vi "Main.vi"(11 "Module Admin":refnum<class "Delacor_lib_QMH_Module Admin.lvclass">) -> ()   [LabVIEW 2024, in "SingletonSubpanel.lvlib"]
doc: "This template is based off of the Queued Message Handler design pattern and the Queued Message Handler project template that ships with LabVIEW.\n\nThe main difference is that the queue is private to this module and communication between modules is performed via Broadcast and Request events.\n\nRequest events are wrapped in public API methods and are handled in the Event Handling Loop (EHL) of this VI. Any module can register for Broadcast events sent by this module. The EHL generates messages based on user interface actions.\n\nThe Message Handling Loop (MHL) processes messages generated by the EHL, or by other messages. The messages are string values, so new messages can be added easily to the Message Cases case structure in the MHL. Each message cluster can also provide an optional value for Message Data, which is a variant that can be converted to whatever message-specific data is required.\n_____\nBased on DQMH Dev Tools: Project Template 7.1.0.1503."
uses:
  SingletonSubpanel.lvlib
  <vilib>/Delacor/Delacor QMH/Libraries/Module Admin_class/Delacor_lib_QMH_Module Admin.lvclass
  Module Data--cluster.ctl
  <vilib>/Delacor/Delacor QMH/Libraries/Message Queue_class/Delacor_lib_QMH_Message Queue.lvclass/Delacor_lib_QMH_Message Queue.ctl
  Stop Argument--cluster.ctl
  <vilib>/Delacor/Delacor QMH/Libraries/Module Admin_class/Delacor_lib_QMH_Module Admin.lvclass/Delacor_lib_QMH_Module Admin.ctl
  Draw FP in Subpanel Argument--cluster.ctl
  Remove From Subpanel Argument--cluster.ctl
  <vilib>/Utility/miscctls.llb/LVPointTypeDef.ctl
  <vilib>/Delacor/Delacor QMH/Libraries/Message Queue_class/Delacor_lib_QMH_Enqueue Message (Single).vi
  <vilib>/Delacor/Delacor QMH/Libraries/Module Admin_class/Delacor_lib_QMH_Get External Launch.vi
  <vilib>/Delacor/Delacor QMH/Libraries/Message Queue_class/Delacor_lib_QMH_Message Queue.lvclass
panel:
  out "error out":errorcluster
  out "Status":string
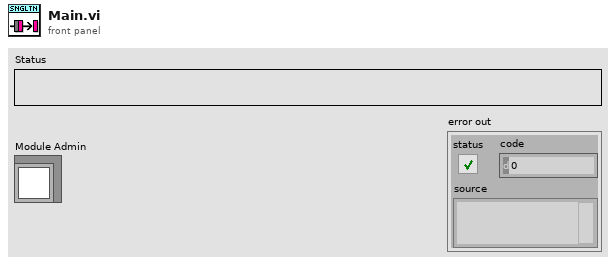
[diagram p1: front panel]
types:
  T1 = typedef "SingletonSubpanel.lvlib/Request Events--cluster.ctl" = cluster{"Stop Module":refnum<user-event>, "Show Panel":refnum<user-event>, "Hide Panel":refnum<user-event>, "Get Module Execution Status":refnum<user-event>, "Show Diagram":refnum<user-event>, "Draw FP in Subpanel":refnum<user-event>, "Remove From Subpanel":refnum<user-event>}
  T2 = typedef "SingletonSubpanel.lvlib/Module Data--cluster.ctl" = cluster{"Status":string, "Sub Panel":refnum<vi>}
  T3 = enum32{"invalid lock state", "Not Locked", "Locked (No Password)", "Password-protected"}
  T4 = typedef "SingletonSubpanel.lvlib/Stop Argument--cluster.ctl" = cluster{"Origin":string, "Exit via Stop Module Req?":bool, "Wait for Module to stop?":bool}
  T5 = typedef "SingletonSubpanel.lvlib/Draw FP in Subpanel Argument--cluster.ctl" = cluster{"Sub Panel":refnum<vi>}
  T6 = typedef "SingletonSubpanel.lvlib/Remove From Subpanel Argument--cluster.ctl" = cluster{"Boolean":bool}
  T7 = typedef "LVPointTypeDef.ctl" = cluster{"Horizontal":i16, "Vertical":i16}
  T8 = enum32{"Invalid", "Standard", "Closed", "Hidden", "Minimized", "Maximized"}
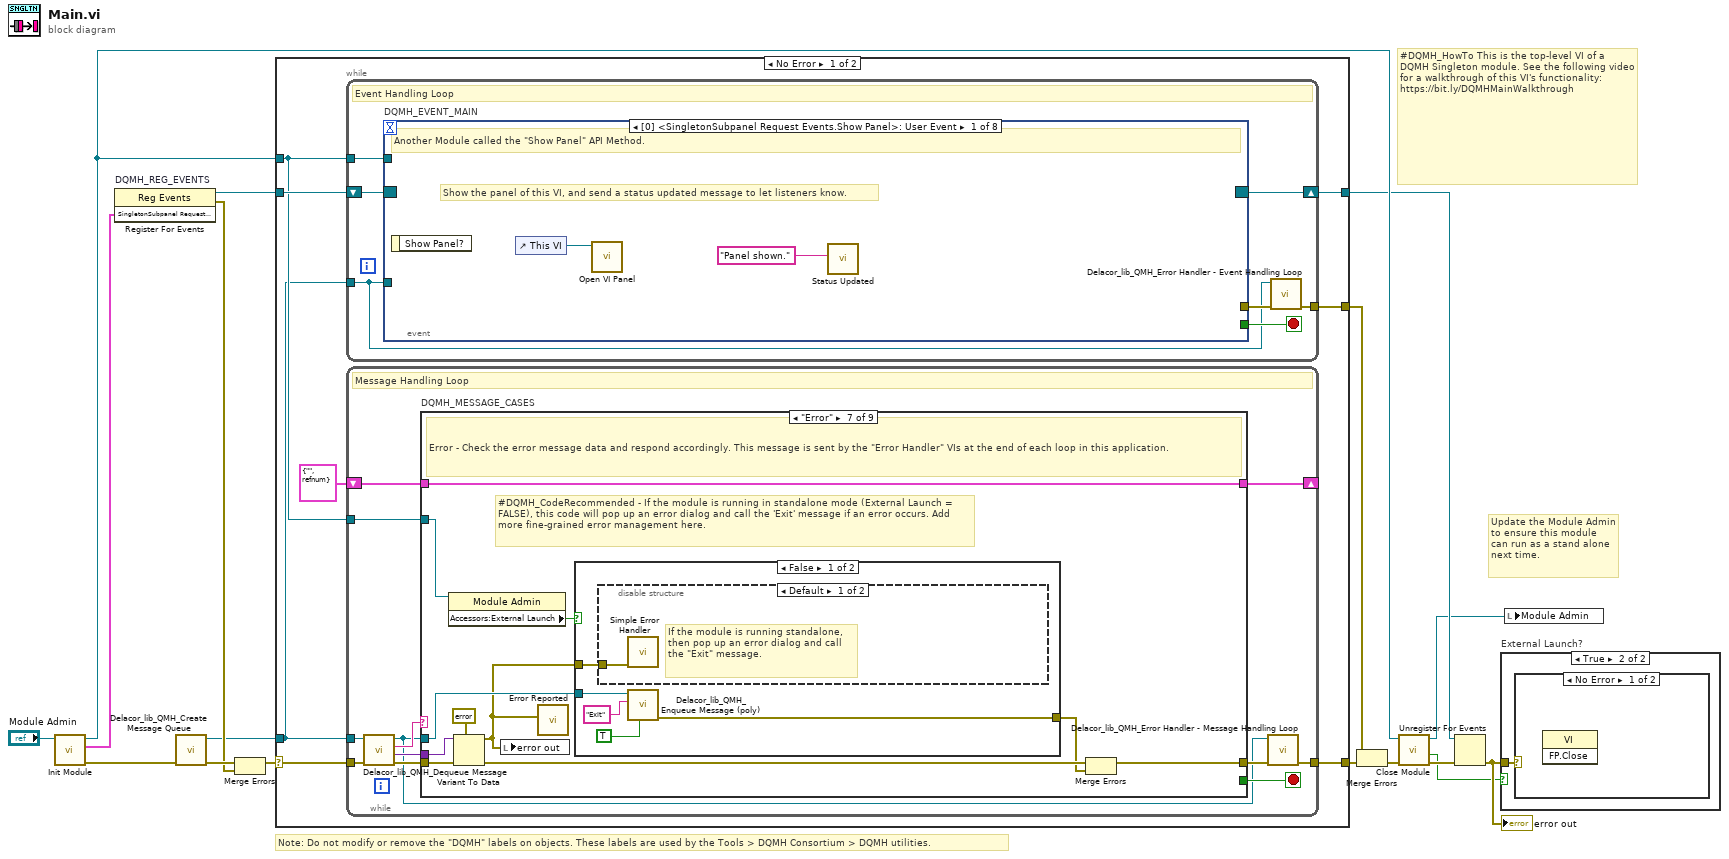
[diagram p0: block diagram]
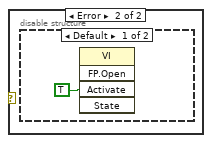
[diagram p3: hidden frame]
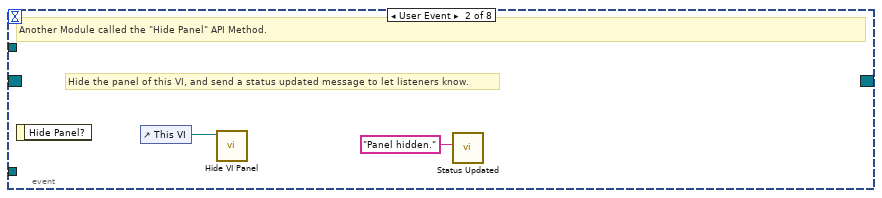
[diagram p5: hidden frame]
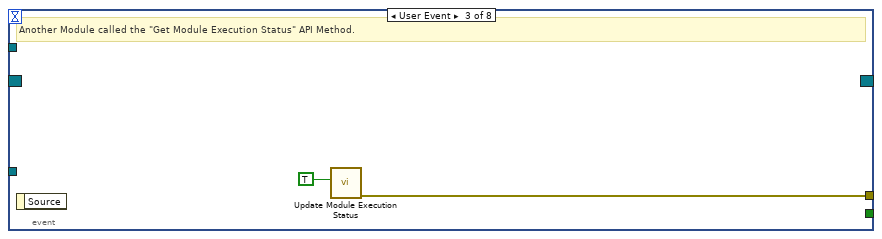
[diagram p6: hidden frame]
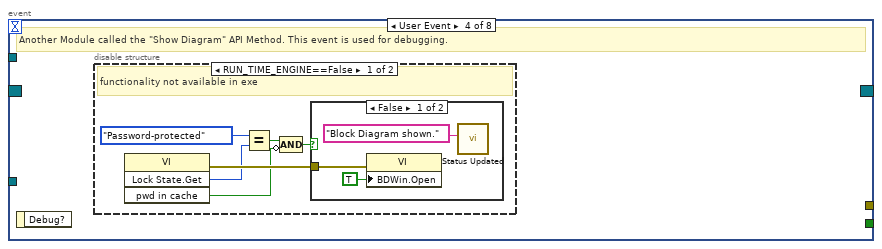
[diagram p7: hidden frame]
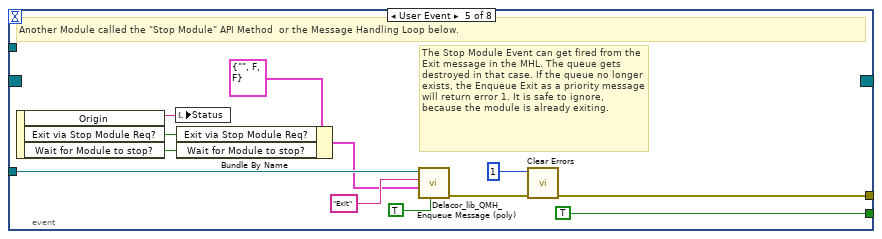
[diagram p10: hidden frame]
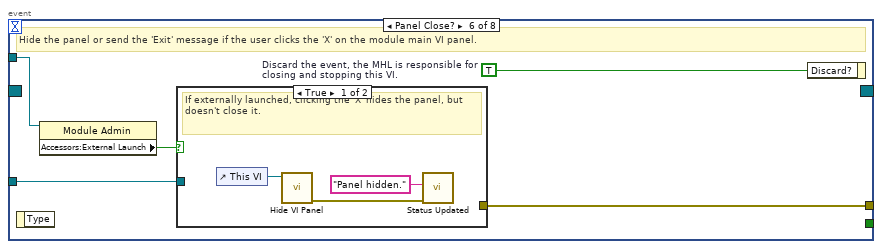
[diagram p11: hidden frame]
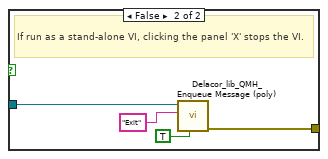
[diagram p12: hidden frame]
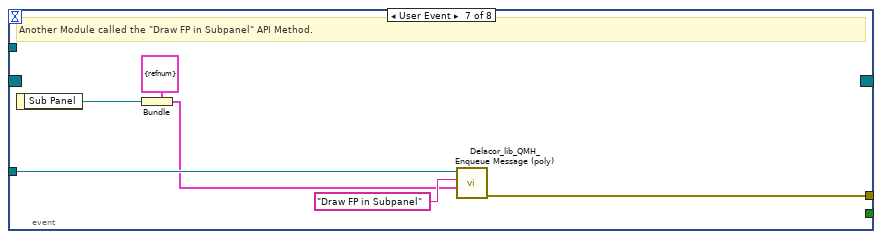
[diagram p13: hidden frame]
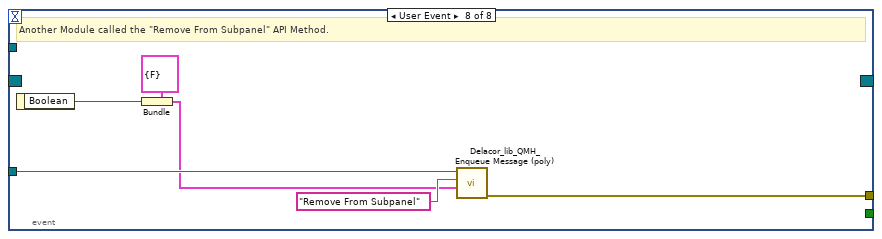
[diagram p14: hidden frame]
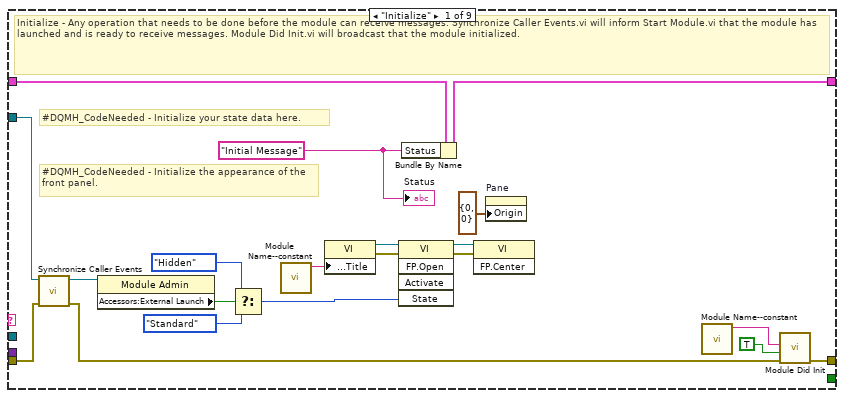
[diagram p15: hidden frame]
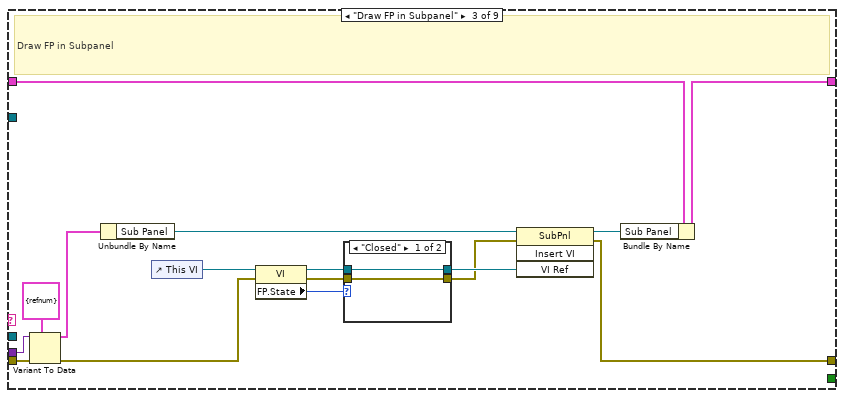
[diagram p17: hidden frame]
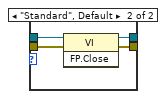
[diagram p18: hidden frame]
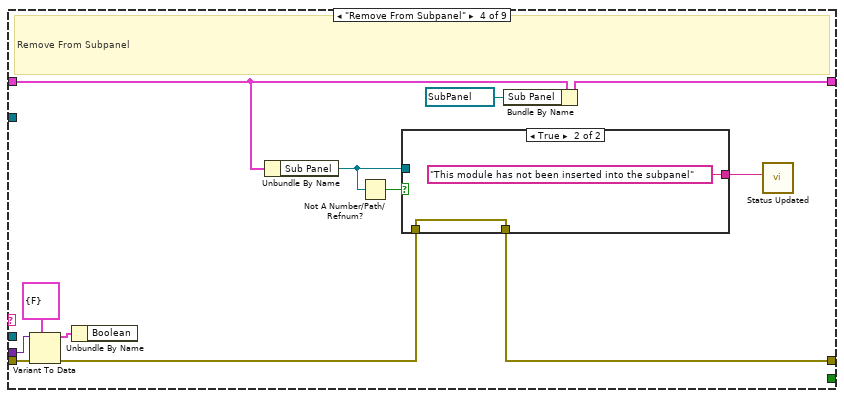
[diagram p19: hidden frame]
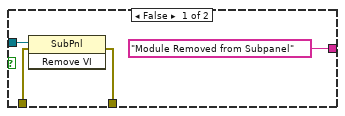
[diagram p20: hidden frame]
diagram:
  # "#DQMH_HowTo This is the top-level VI of a DQMH Singleton module. See the following video for a walkthrough of this VI's functionality: https://bit.ly/DQMHMainWalkthrough"
  # "Note: Do not modify or remove the \"DQMH\" labels on objects. These labels are used by the Tools > DQMH Consortium > DQMH utilities."
  # "Update the Module Admin to ensure this module can run as a stand alone next time."
  n1 = call "Init Module.vi"("Singleton Module Admin in"="Module Admin") -> ("error out"=w16:errorcluster, "SingletonSubpanel Request Events"=w5:T1, "Singleton Module Admin out"=w8:refnum<class "Delacor_lib_QMH_Module Admin.lvclass">)  [unwired: 8 in]
  n2 = register-events "DQMH_REG_EVENTS"(w5) -> (reference out=w6:refnum<event-registration>, error out=w9:errorcluster)  [unwired: 2 in]
  n3 = call <vilib>:"Delacor_lib_QMH_Create Message Queue.vi"("error in"=w16) -> ("error out"=w11:errorcluster, "Message Queue"=w4:refnum<class "Delacor_lib_QMH_Message Queue.lvclass">)  [unwired: 9 in]
  n4 = Merge Errors(w11, w9) -> (w10:errorcluster)
  n5 = case shown="No Error" w10 {
    selector: w10 -> [w23 w213]
    tunnel: [w25 w212] -> w17
    tunnel: [w22 w211] -> w7
    tunnel: w6 -> [w20 w211]
    tunnel: w4 -> [w18 w206]
    tunnel: [w24 _] -> w14
    tunnel: w8 -> [w19 w207]
    frame No Error {
      n6 = while {
        tunnel: w18 -> [w26]
        shift-right: [w29] -> w22
        shift-left: w20 -> [w30]
        tunnel: [w31] -> w24
        tunnel: w19 -> [w27]
        stop <- w28 stop-if-true
        # "Event Handling Loop"
        n7 = event "DQMH_EVENT_MAIN" shown="[0] <SingletonSubpanel Request Events.Show Panel>: User Event" {
          selector: w30 -> [_ _ _ _ _ _ _ _]
          dyn-events: [_ _ _ _ _ _ _ _] -> w29
          timeout: _ -> [_ _ _ _ _ _ _ _]
          tunnel: [_ _ _ _ TRUE ("Discard?") _ _ _] -> w28
          tunnel: w26 -> [_ _ _ _ w55 w62 w77 w83]
          tunnel: [_ _ w38 _ w58 w64 w72 w78] -> w32
          tunnel: w27 -> [_ _ _ _ _ w61 _ _]
          event User Event {
            # "Show the panel of this VI, and send a status updated message to let listeners know."
            # "Another Module called the \"Show Panel\" API Method."
            n8 = event-data() -> ()  [unwired: 1 in, 1 out]
            n9 = control-ref of="This VI"() -> (w34:refnum<vi>)
            n10 = call "Open VI Panel.vi"("VI"=w34) -> ()  [unwired: 10 in, 1 out]
            n11 = call "Status Updated.vi"("Status"="Panel shown." ("format string")) -> ()  [unwired: 10 in, 1 out]
          }
          event User Event {
            # "Hide the panel of this VI, and send a status updated message to let listeners know."
            # "Another Module called the \"Hide Panel\" API Method."
            n12 = event-data() -> ()  [unwired: 1 in, 1 out]
            n13 = control-ref of="This VI"() -> (w36:refnum<vi>)
            n14 = call "Hide VI Panel.vi"("VI"=w36) -> ()  [unwired: 10 in, 1 out]
            n15 = call "Status Updated.vi"("Status"="Panel hidden." ("format string")) -> ()  [unwired: 10 in, 1 out]
          }
          event User Event {
            # "Another Module called the \"Get Module Execution Status\" API Method."
            n16 = event-data() -> ()  [unwired: 1 in, 1 out]
            n17 = call "Update Module Execution Status.vi"("Running?"=TRUE) -> ("error out"=w38:errorcluster)  [unwired: 10 in]
          }
          event User Event {
            # "Another Module called the \"Show Diagram\" API Method. This event is used for debugging."
            n18 = event-data() -> ()  [unwired: 1 in, 1 out]
            n19 = disable-structure shown="RUN_TIME_ENGINE==False" {
              frame condition #0 (active) {
                # "functionality not available in exe"
                n20 = invoke on="Invoke Node" class="VI" method="Lock State.Get"() -> (error out=w44:errorcluster, "Get Lock State"=w43:T3, "pwd in cache"=w40:bool)  [unwired: 4 in, 1 out]
                n21 = Equal?(x=T3."Password-protected", y=w43) -> (x = y?=w41:bool)
                n22 = Compound Arithmetic op=AND(w41, invert w40) -> (w39:bool)
                n23 = case shown="False" w39 {
                  tunnel: w44 -> [w47 _]
                  frame False {
                    n24 = property on="Property Node" class="VI"(error in=w47, "BDWin.Open"=TRUE ("Block Diagram Window:Open")) -> ()  [unwired: 1 in, 2 out]
                    n25 = call "Status Updated.vi"("Status"="Block Diagram shown." ("format string")) -> ()  [unwired: 10 in, 1 out]
                  }
                  frame True {
                    # "Password-protected VI, and the password is not in the cache. Do not show the diagram."
                  }
                }
              }
              frame condition #1 {
              }
            }
          }
          event User Event {
            # "The Stop Module Event can get fired from the Exit message in the MHL. The queue gets destroyed in that case. If the queue no longer exists, the Enqueue Exit as a priority message will return error 1. It is safe to ignore, because the module is already exiting."
            # "Another Module called the \"Stop Module\" API Method  or the Message Handling Loop below."
            n26 = event-data() -> ("Origin"=w54:string, "Exit via Stop Module Req?"=w50:bool, "Wait for Module to stop?"=w49:bool)  [unwired: 1 in]
            n27 = local write "Status"(w54) -> ()
            n28 = Bundle By Name(cluster=T4 {"Origin"="", "Exit via Stop Module Req?"=FALSE, "Wait for Module to stop?"=FALSE} ("Stop Argument"), "Exit via Stop Module Req?"=w50, "Wait for Module to stop?"=w49) -> (w48:T4)
            n29 = call-poly <vilib>:"Delacor_lib_QMH_Enqueue Message (poly).vi"("Priority Message? (F)"=TRUE, "Message Data"=w48, "Message"="Exit", "Message Queue in"=w55) -> ("error out"=w59:errorcluster)  [unwired: 6 in, 1 out]
            n30 = call <vilib>:"Clear Errors.vi"("error in (no error)"=w59, "specific error code to clear (0: all)"=1) -> ("error out"=w58:errorcluster)  [unwired: 4 in, 1 out]
          }
          event Panel Close? {
            w63 = TRUE  # Discard the event, the MHL is responsible for closing and stopping this VI.
            # "Hide the panel or send the 'Exit' message if the user clicks the 'X' on the module main VI panel."
            n31 = event-data() -> ()  [unwired: 1 in, 1 out]
            n32 = property on="Property Node" class="Module Admin"(reference=w61) -> ("Accessors:External Launch"=w60:bool)  [unwired: 1 in, 2 out]
            n33 = case shown="True" w60 {
              tunnel: w62 -> [_ w70]
              tunnel: [_ w71] -> w64
              frame True {
                # "If externally launched, clicking the 'X' hides the panel, but doesn't close it."
                n34 = control-ref of="This VI"() -> (w67:refnum<vi>)
                n35 = call "Hide VI Panel.vi"("VI"=w67) -> ("error out"=w65:errorcluster)  [unwired: 10 in]
                n36 = call "Status Updated.vi"("error in"=w65, "Status"="Panel hidden." ("format string")) -> ()  [unwired: 9 in, 1 out]
              }
              frame False {
                # "If run as a stand-alone VI, clicking the panel 'X' stops the VI."
                n37 = call-poly <vilib>:"Delacor_lib_QMH_Enqueue Message (poly).vi"("Priority Message? (F)"=TRUE, "Message"="Exit", "Message Queue in"=w70) -> ("error out"=w71:errorcluster)  [unwired: 7 in, 1 out]
              }
            }
            n38 = event-data ("Event Filter Node")("Discard?"=w63) -> ()  [unwired: 1 in, 1 out]
          }
          event User Event {
            # "Another Module called the \"Draw FP in Subpanel\" API Method."
            n39 = event-data() -> ("Sub Panel"=w73:refnum<vi>)  [unwired: 1 in]
            n40 = Bundle(cluster=T5 {"Sub Panel"=refnum} ("Draw FP in Subpanel Argument"), "Sub Panel"=w73) -> (w74:T5)
            n41 = call-poly <vilib>:"Delacor_lib_QMH_Enqueue Message (poly).vi"("Message Data"=w74, "Message"="Draw FP in Subpanel", "Message Queue in"=w77) -> ("error out"=w72:errorcluster)  [unwired: 7 in, 1 out]
          }
          event User Event {
            # "Another Module called the \"Remove From Subpanel\" API Method."
            n42 = event-data() -> ("Boolean"=w79:bool)  [unwired: 1 in]
            n43 = Bundle(cluster=T6 {"Boolean"=FALSE} ("Remove From Subpanel Argument"), "Boolean"=w79) -> (w80:T6)
            n44 = call-poly <vilib>:"Delacor_lib_QMH_Enqueue Message (poly).vi"("Message Data"=w80, "Message"="Remove From Subpanel", "Message Queue in"=w83) -> ("error out"=w78:errorcluster)  [unwired: 7 in, 1 out]
          }
        }
        n45 = call-dynamic "Delacor_lib_QMH_Error Handler - Event Handling Loop.vi"("error in"=w32, "Message Queue in"=w26) -> ("dup error in"=w31:errorcluster)  [unwired: 8 in, 1 out]
      }
      n46 = while {
        tunnel: w18 -> [w84]
        shift-right: [w92] -> _
        shift-left: T2 {"Status"="", "Sub Panel"=refnum} ("Data Cluster") -> [w93]
        tunnel: w23 -> [w95]
        tunnel: [w87] -> w25
        tunnel: w19 -> [w88]
        stop <- w91 stop-if-true
        # "Message Handling Loop"
        n47 = call-dynamic "Delacor_lib_QMH_Dequeue Message.vi"("error in"=w95, "Message Queue in"=w84) -> ("error out"=w94:errorcluster, "Message Data"=w89:variant, "Message"=w90:string, "Message Queue out"=w85:refnum<class "Delacor_lib_QMH_Message Queue.lvclass">)  [unwired: 6 in]
        n48 = case "DQMH_MESSAGE_CASES" shown="\"Error\"" w90 {
          selector: w90 -> [_ _ _ _ _ _ _ _ w201]
          tunnel: w85 -> [_ _ _ _ _ _ w166 w189 _]
          tunnel: w94 -> [w113 w117 w133 w151 w160 w162 w173 w195 w204]
          tunnel: [w111 w117 w125 w145 w159 w162 w169 w190 w205] -> w86
          tunnel: w93 -> [w102 w116 w132 w147 w158 w161 w168 w181 w202]
          tunnel: [w101 w116 w128 w142 w158 w161 w168 w181 w202] -> w92
          tunnel: [_ _ _ _ _ _ _ w188 _] -> w91
          tunnel: w89 -> [_ _ w131 w150 _ _ w167 w187 _]
          tunnel: w88 -> [w103 _ _ _ _ _ w165 w182 _]
          frame "Initialize" {
            w97 = "Initial Message" ("Initial Message")
            # "#DQMH_CodeNeeded - Initialize the appearance of the front panel."
            # "#DQMH_CodeNeeded - Initialize your state data here."
            # "Initialize - Any operation that needs to be done before the module can receive messages. Synchronize Caller Events.vi will inform Start Module.vi that the module has launched and is ready to receive messages. Module Did Init.vi will broadcast that the module initialized."
            n49 = call "Synchronize Caller Events.vi"("error in"=w113, "Singleton Module Admin in"=w103) -> ("error out"=w112:errorcluster, "Singleton Module Admin out"=w98:refnum<class "Delacor_lib_QMH_Module Admin.lvclass">)  [unwired: 8 in]
            n50 = property on="Property Node" class="Module Admin"(reference=w98) -> ("Accessors:External Launch"=w107:bool)  [unwired: 1 in, 2 out]
            n51 = Select(t=T8."Hidden" ("State"), s=w107, f=T8."Standard" ("State")) -> (s? t:f=w104:T8)
            n52 = call "Module Name--constant.vi"() -> ("Module Name"=w110:string)  [unwired: 11 in]
            n53 = property on="Property Node" class="VI"("Front Panel.Title"=w110) -> (reference out=w109:refnum<vi>, error out=w115:errorcluster)  [unwired: 2 in]
            n54 = invoke on="Invoke Node" class="VI" method="FP.Open"(reference=w109, error in=w115, "State"=w104) -> (reference out=w108:refnum<vi>, error out=w114:errorcluster)  [unwired: 2 in, 3 out]
            n55 = Bundle By Name(cluster=w102, "Status"=w97) -> (w101:T2)
            n56 = invoke on="Invoke Node" class="VI" method="FP.Center"(reference=w108, error in=w114) -> ()  [unwired: 1 in, 3 out]
            n57 = property on="Pane" class="Pane"("Origin"=T7 {"Horizontal"=0, "Vertical"=0}) -> ()  [unwired: 2 in, 2 out]
            n58 = call "Module Name--constant.vi"() -> ("Module Name"=w99:string)  [unwired: 11 in]
            n59 = call "Module Did Init.vi"("error in"=w112, "Initialized?"=TRUE, "Origin"=w99) -> ("error out"=w111:errorcluster)  [unwired: 8 in]
            "Status" <- w97
          }
          frame "---Module Specific---" {
            # "Separator -- The following cases handle messages specific to this Module."
          }
          frame "Draw FP in Subpanel" {
            # "Draw FP in Subpanel"
            n60 = Variant To Data(error in=w133, type=T5 {"Sub Panel"=refnum} ("Draw FP in Subpanel Argument"), Variant=w131) -> (data=w129:T5, error out=w123:errorcluster)
            n61 = Unbundle By Name(w129) -> ("Sub Panel"=w127:refnum<vi>)
            n62 = control-ref of="This VI"() -> (w120:refnum<vi>)
            n63 = property class="VI"(reference=w120, error in=w123) -> (reference out=w119:refnum<vi>, error out=w121:errorcluster, "FP.State"=w118:T8)
            n64 = case shown="\"Closed\"" w118 {
              tunnel: [w135 w139] -> w124
              tunnel: [w134 w138] -> w122
              tunnel: w121 -> [w134 w137]
              tunnel: w119 -> [w135 w136]
              frame "Closed" {
              }
              frame "Standard", Default {
                n65 = invoke class="VI" method="FP.Close"(reference=w136, error in=w137) -> (reference out=w139:refnum<vi>, error out=w138:errorcluster)  [unwired: 1 in, 1 out]
              }
            }
            n66 = invoke class="SubPnl" method="Insert VI"(reference=w127, error in=w122, "VI Ref"=w124) -> (reference out=w126:refnum<vi>, error out=w125:errorcluster)  [unwired: 1 in, 2 out]
            n67 = Bundle By Name(cluster=w132, "Sub Panel"=w126) -> (w128:T2)
          }
          frame "Remove From Subpanel" {
            # "Remove From Subpanel"
            n68 = Variant To Data(error in=w151, type=T6 {"Boolean"=FALSE} ("Remove From Subpanel Argument"), Variant=w150) -> (data=w148:T6, error out=w146:errorcluster)
            n69 = Unbundle By Name(w148) -> ()  [unwired: 1 out]
            n70 = Unbundle By Name(w147) -> ("Sub Panel"=w144:refnum<vi>)
            n71 = Not A Number/Path/Refnum?(number/path/refnum=w144) -> (NaN/Path/Refnum?=w143:bool)
            n72 = case shown="True" w143 {
              tunnel: w146 -> [w155 w157]
              tunnel: [w154 w157] -> w145
              tunnel: w144 -> [w153 _]
              tunnel: ["Module Removed from Subpanel" "This module has not been inserted into the subpanel"] -> w140
              frame False {
                n73 = invoke class="SubPnl" method="Remove VI"(reference=w153, error in=w155) -> (error out=w154:errorcluster)  [unwired: 1 in, 2 out]
              }
              frame True {
              }
            }
            n74 = Bundle By Name(cluster=w147, "Sub Panel"=refnum<vi> refnum) -> (w142:T2)
            n75 = call "Status Updated.vi"("Status"=w140) -> ()  [unwired: 10 in, 1 out]
          }
          frame "---Copy This Frame---" {
            # "Duplicate this frame when creating new messages.  Change this comment in the duplicated frame to describe this message."
            n76 = Merge Errors(w160) -> (w159:errorcluster)
          }
          frame "---Exit and Error Handling---" {
            # "Separator - The following cases handle errors and exit messages."
          }
          frame "Error" {
            # "#DQMH_CodeRecommended - If the module is running in standalone mode (External Launch = FALSE), this code will pop up an error dialog and call the 'Exit' message if an error occurs. Add more fine-grained error management here."
            # "Error - Check the error message data and respond accordingly. This message is sent by the \"Error Handler\" VIs at the end of each loop in this application."
            n77 = property on="Property Node" class="Module Admin"(reference=w165) -> ("Accessors:External Launch"=w164:bool)  [unwired: 1 in, 2 out]
            n78 = Variant To Data(error in=w173, type=errorcluster {"status"=FALSE, "code"=0, "source"=""} ("error constant"), Variant=w167) -> (data=w163:errorcluster, error out=w171:errorcluster)
            n79 = local write "error out"(w163) -> ()
            n80 = call "Error Reported.vi"("Error"=w163) -> ()  [unwired: 10 in, 1 out]
            n81 = case shown="False" w164 {
              tunnel: [w178 _] -> w170
              tunnel: w166 -> [w176 _]
              tunnel: w163 -> [w177 _]
              frame False {
                n82 = disable-structure shown="Default" {
                  disable-tunnel: w177 -> [w179 _]
                  frame condition #0 (active) {
                    # "If the module is running standalone, then pop up an error dialog and call the \"Exit\" message."
                    n83 = call <vilib>:"Simple Error Handler.vi"("error in (no error)"=w179) -> ()  [unwired: 4 in, 5 out]
                  }
                  frame condition #1 {
                    # "To prevent the Simple Error Handler VI from being loaded (e.g. when deploying to a Real-Time target), add the Conditional Disable Symbol \"DQMH_Disable_SEH\" to your project and set it to TRUE."
                  }
                }
                n84 = call-poly <vilib>:"Delacor_lib_QMH_Enqueue Message (poly).vi"("Priority Message? (F)"=TRUE, "Message"="Exit", "Message Queue in"=w176) -> ("error out"=w178:errorcluster)  [unwired: 7 in, 1 out]
              }
              frame True {
                # "If the module was launched externally, calling the Error Reported broadcast VI is the only action performed by the \"Error\" message. The module's caller can then process the error appropriately."
              }
            }
            n85 = Merge Errors(w171, w170) -> (w169:errorcluster)
          }
          frame "Exit" {
            w186 = 91  # 91: not all Exit messages will have an argument
            w188 = TRUE  # Stop the VI
            # "Release the message queue reference"
            # "#DQMH_CodeNeeded - Add any required cleanup code here."
            # "Exit - Exit the application."
            n86 = Variant To Data(error in=w195, type=T4 {"Origin"="", "Exit via Stop Module Req?"=FALSE, "Wait for Module to stop?"=FALSE} ("Stop Argument"), Variant=w187) -> (data=w184:T4, error out=w192:errorcluster)
            n87 = call <vilib>:"Clear Errors.vi"("error in (no error)"=w192, "specific error code to clear (0: all)"=w186) -> ("error out"=w194:errorcluster)  [unwired: 4 in, 1 out]
            n88 = control-ref of="This VI"() -> (w183:refnum<vi>)
            n89 = call-dynamic "Delacor_lib_QMH_Release Message Queue.vi"("error in"=w194, "Message Queue"=w189) -> ("error out"=w193:errorcluster)  [unwired: 9 in]
            n90 = call "Handle Exit.vi"("Stop Argument"=w184, "Admin in"=w182, "VI reference"=w183) -> ("error out"=w191:errorcluster)  [unwired: 7 in, 1 out]
            n91 = Merge Errors(w193, w191) -> (w190:errorcluster)
            n92 = Unbundle By Name(w181) -> ("Sub Panel"=w180:refnum<vi>)
            n93 = call "Error Reported.vi"("Error"=w190) -> ()  [unwired: 10 in, 1 out]
            n94 = invoke class="SubPnl" method="Remove VI"(reference=w180) -> ()  [unwired: 2 in, 3 out]
          }
          frame Default {
            # "'Default' case only runs if there is a message that isn't defined in any of the other cases.  Output a programming error."
            n95 = call "Module Name--constant.vi"() -> ("Module Name"=w200:string)  [unwired: 11 in]
            n96 = Format Into String(format string="The invalid message string \"%s\" was received in the Message Handling Loop for module \"%s\".", w201, w200) -> (resulting string=w196:string)  [unwired: 2 in, 1 out]
            n97 = call <vilib>:"Error Cluster From Error Code.vi"("show call chain? (False)"=TRUE, "error message (\"\")"=w196, "error code (0)"=1) -> ("error out"=w203:errorcluster)  [unwired: 6 in]
            n98 = Merge Errors(w204, w203) -> (w205:errorcluster)
          }
        }
        n99 = call-dynamic "Delacor_lib_QMH_Error Handler - Message Handling Loop.vi"("error in"=w86, "Message Queue in"=w85) -> ("dup error in"=w87:errorcluster)  [unwired: 8 in, 1 out]
      }
    }
    frame Error {
      # "Synchronize Caller Events.vi will inform Start Module.vi that the module has launched and will let the code calling Start Module.vi register for broadcasts and would permit the caller receive the broadcast that an error occurred at launch time."
      n100 = call-dynamic "Delacor_lib_QMH_Release Message Queue.vi"("error in"=w213, "Message Queue"=w206) -> ("error out"=w212:errorcluster)  [unwired: 9 in]
      n101 = call "Synchronize Caller Events.vi"("Singleton Module Admin in"=w207) -> ("error out"=w214:errorcluster)  [unwired: 9 in, 1 out]
      n102 = call "Module Name--constant.vi"() -> ("Module Name"=w210:string)  [unwired: 11 in]
      n103 = Format Into String(format string="An error occurred during initialization. %s is no longer running.", w210) -> (resulting string=w208:string)  [unwired: 2 in, 1 out]
      n104 = Merge Errors(w212, w214) -> (w215:errorcluster)
      n105 = call "Error Reported.vi"("Additional Information"=w208, "Error"=w215) -> ()  [unwired: 9 in, 1 out]
    }
  }
  n106 = Merge Errors(w14, w17) -> (w13:errorcluster)
  n107 = call "Close Module.vi"("error in"=w13, "Module Admin in"=w8) -> ("error out"=w15:errorcluster, "External Launch"=w1:bool, "Module Admin out"=w2:refnum<class "Delacor_lib_QMH_Module Admin.lvclass">)  [unwired: 7 in]
  n108 = Unregister For Events(event registration refnum=w7, error in=w15) -> (error out=w12:errorcluster)
  "error out" <- w12
  n109 = case "External Launch?" shown="True" w1 {
    tunnel: w12 -> [_ w216]
    frame False {
    }
    frame True {
      n110 = case shown="No Error" w216 {
        frame No Error {
          n111 = invoke on="Invoke Node" class="VI" method="FP.Close"() -> ()  [unwired: 3 in, 3 out]
        }
        frame Error {
          n112 = disable-structure shown="Default" {
            frame condition #0 (active) {
              n113 = invoke class="VI" method="FP.Open"("Activate"=TRUE ("Activate?")) -> ()  [unwired: 4 in, 5 out]
            }
            frame condition #1 {
              # "Don't show panel on error if running inside a built EXE."
            }
          }
        }
      }
    }
  }
  n114 = local write "Module Admin"(w2) -> ()
